vi "Unflatten Value.vi"(8 "error in (no error)":errorcluster, 10 "Value":string, 11 "Boolean in":refnum<class "Test Executive.lvclass">) -> (0 "error out":errorcluster, 3 "Boolean out":refnum<class "Test Executive.lvclass">)   [LabVIEW 2017, in "Custom Type Test Executive.lvlib" / "Test Executive.lvclass"]
uses:
  <vilib>/gpm_packages/@cs/test-executive/Source/Custom Type Test Executive/Test Executive Data Type/Test Executive.lvclass
  <vilib>/gpm_packages/@cs/test-executive/Source/Test Executive/ITestExecutive/ITest Executive.lvclass
  <vilib>/gpm_packages/@cs/test-executive/Source/Custom Type Test Executive/Test Executive Data Type/Test Executive.lvclass/Test Executive.ctl
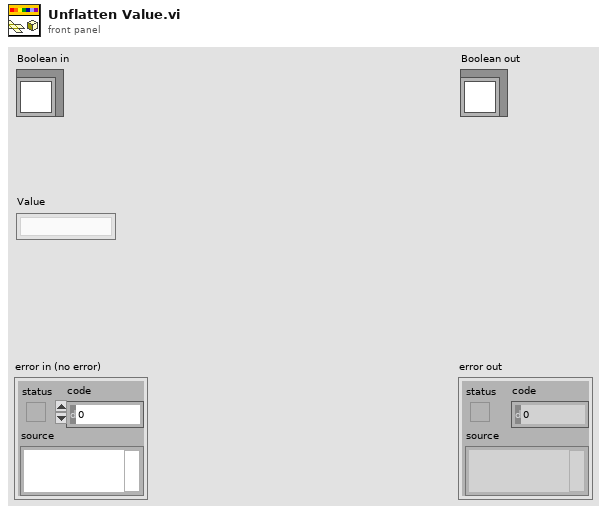
[diagram p1: front panel]
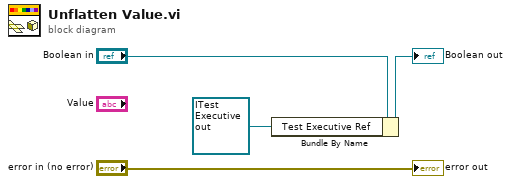
[diagram p0: block diagram]
diagram:
  n1 = Bundle By Name(cluster="Boolean in", "Test Executive Ref"=refnum<data-value> refnum) -> (→"Boolean out":refnum<class "Test Executive.lvclass">)
  "error out" <- "error in (no error)"
